vi "InterruptOccuranceGenerator.vi"() -> (0 "Occurances":T1)   [LabVIEW 2019]
uses:
  Controls/Interrupt_Occurances.ctl
  <vilib>/rvi/Emulation/niFpgaSctlEmulationGetInTimedLoop.vi
  <vilib>/rvi/Emulation/niFpgaProcessEmulError.vi
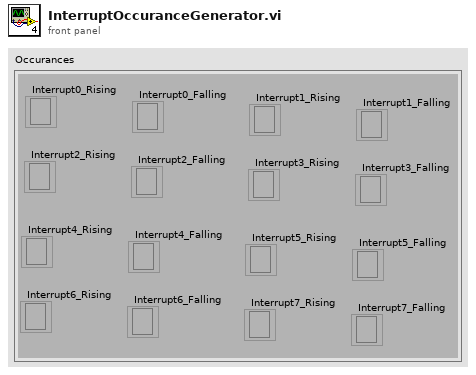
[diagram p1: front panel]
types:
  T1 = typedef "Interrupt_Occurances.ctl" = cluster{"Interrupt0_Rising":refnum<k4>, "Interrupt0_Falling":refnum<k4>, "Interrupt1_Rising":refnum<k4>, "Interrupt1_Falling":refnum<k4>, "Interrupt2_Rising":refnum<k4>, "Interrupt2_Falling":refnum<k4>, "Interrupt3_Rising":refnum<k4>, "Interrupt3_Falling":refnum<k4>, "Interrupt4_Rising":refnum<k4>, "Interrupt4_Falling":refnum<k4>, "Interrupt5_Rising":refnum<k4>, "Interrupt5_Falling":refnum<k4>, "Interrupt6_Rising":refnum<k4>, "Interrupt6_Falling":refnum<k4>, "Interrupt7_Rising":refnum<k4>, "Interrupt7_Falling":refnum<k4>}
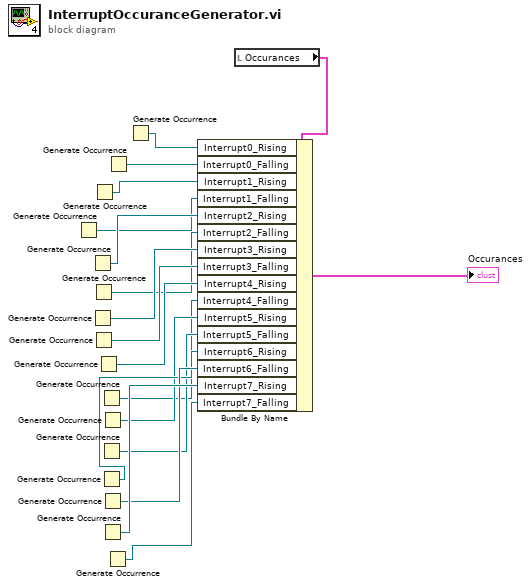
[diagram p0: block diagram]
diagram:
  n1 = Generate Occurrence() -> (w6:refnum<k4>)
  n2 = Generate Occurrence() -> (w7:refnum<k4>)
  n3 = Generate Occurrence() -> (w9:refnum<k4>)
  n4 = Generate Occurrence() -> (w8:refnum<k4>)
  n5 = Generate Occurrence() -> (w10:refnum<k4>)
  n6 = Generate Occurrence() -> (w5:refnum<k4>)
  n7 = Generate Occurrence() -> (w11:refnum<k4>)
  n8 = Generate Occurrence() -> (w12:refnum<k4>)
  n9 = Generate Occurrence() -> (w14:refnum<k4>)
  n10 = Generate Occurrence() -> (w15:refnum<k4>)
  n11 = Generate Occurrence() -> (w13:refnum<k4>)
  n12 = Generate Occurrence() -> (w16:refnum<k4>)
  n13 = Generate Occurrence() -> (w17:refnum<k4>)
  n14 = Generate Occurrence() -> (w18:refnum<k4>)
  n15 = Generate Occurrence() -> (w4:refnum<k4>)
  n16 = Generate Occurrence() -> (w3:refnum<k4>)
  n17 = local read "Occurances"() -> (w1:T1)
  n18 = Bundle By Name(cluster=w1, "Interrupt0_Rising"=w3, "Interrupt0_Falling"=w4, "Interrupt1_Rising"=w5, "Interrupt1_Falling"=w6, "Interrupt2_Rising"=w7, "Interrupt2_Falling"=w8, "Interrupt3_Rising"=w9, "Interrupt3_Falling"=w10, "Interrupt4_Rising"=w11, "Interrupt4_Falling"=w12, "Interrupt5_Rising"=w13, "Interrupt5_Falling"=w14, "Interrupt6_Rising"=w15, "Interrupt6_Falling"=w16, "Interrupt7_Rising"=w17, "Interrupt7_Falling"=w18) -> (→"Occurances":T1)
